vi "Configuration UI.vi"(0 "Engine":refnum<k7>, 5 "Data In":T1, 7 "Sequence Context In":refnum<k7>, 11 "error in (no error)":errorcluster) -> (4 "Engine out":refnum<k7>, 6 "Data Out":T1, 8 "Changed":bool, 15 "error out":errorcluster)   [LabVIEW 2019, in "STS_LTRV.lvlib"]
uses:
  STS_LTRV.lvlib
  TypeDefs/Config UI Data Type.ctl
  SimpleTextPlugin.llb/SimpleTextRpt - TestStand - End Modal Dialog (Engine).vi
  SimpleTextPlugin.llb/SimpleTextRpt - TestStand - Start Modal Dialog (Engine).vi
panel:
  in  "Max UUT Records to Store":u32=4 min=4
  in  "TS_HELP":bool
  in  "TS_CANCEL":bool
  in  "TS_OK":bool
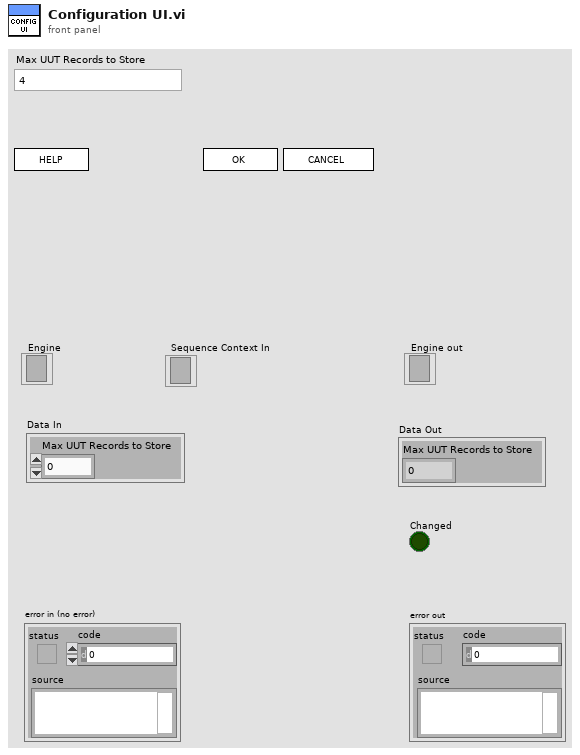
[diagram p1: front panel]
types:
  T1 = typedef "STS_LTRV.lvlib/Config UI Data Type.ctl" = cluster{"Max UUT Records to Store":u32}
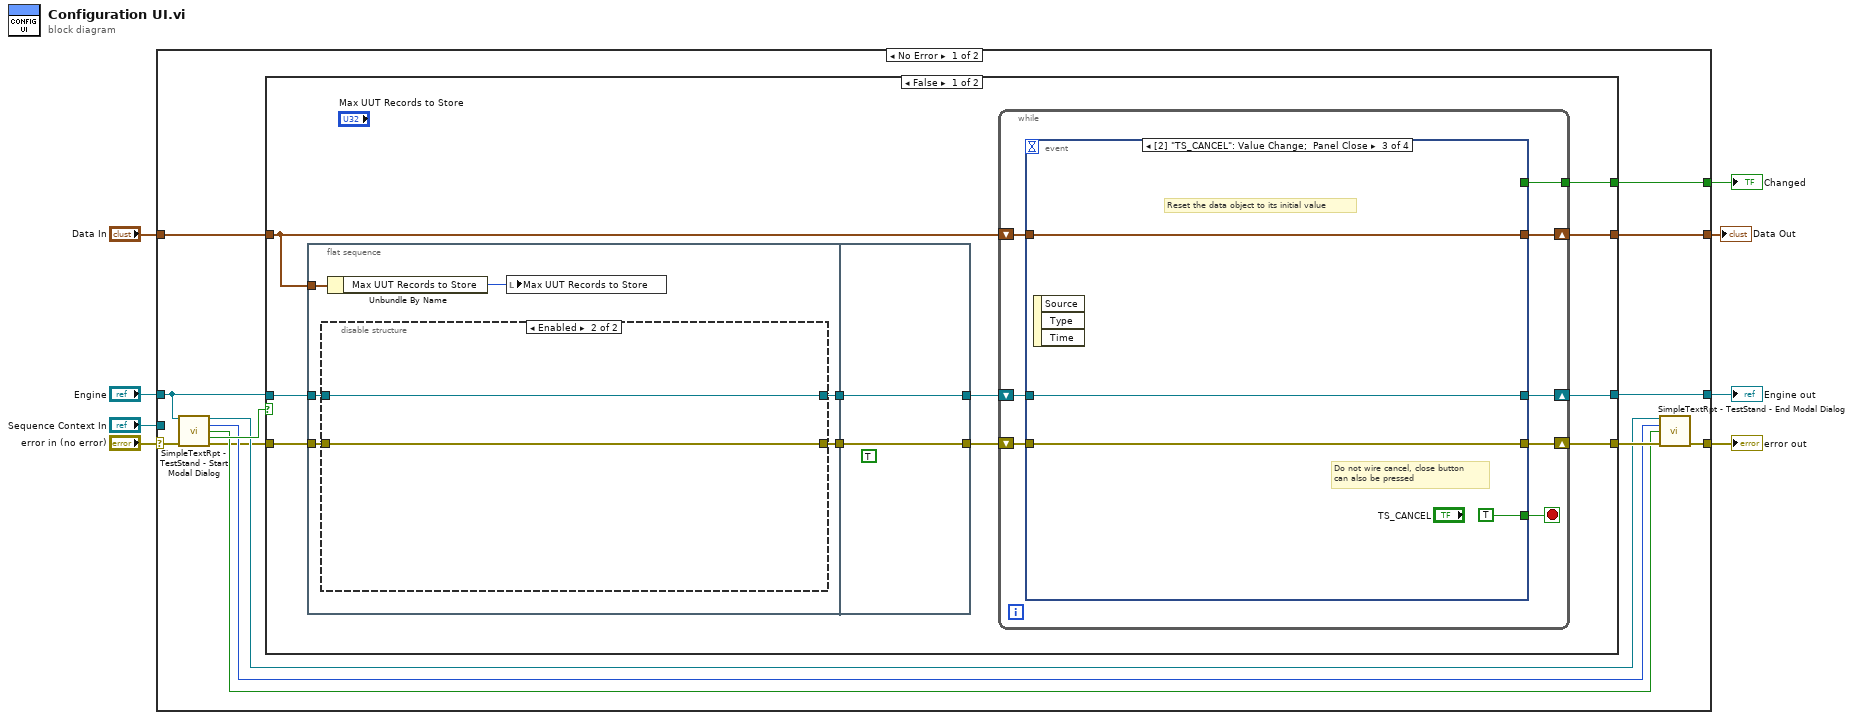
[diagram p0: block diagram]
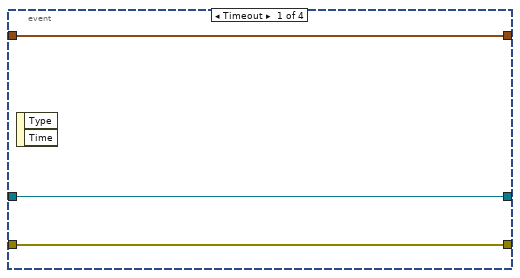
[diagram p2: hidden frame]
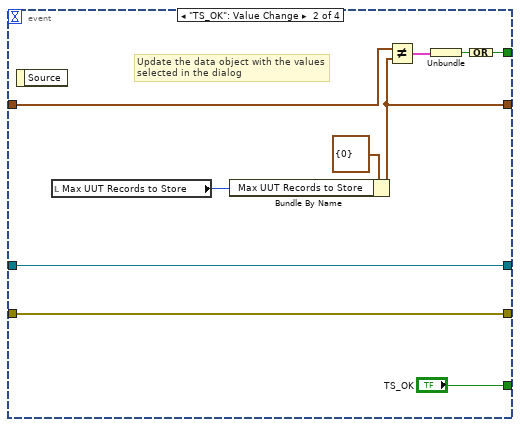
[diagram p3: hidden frame]
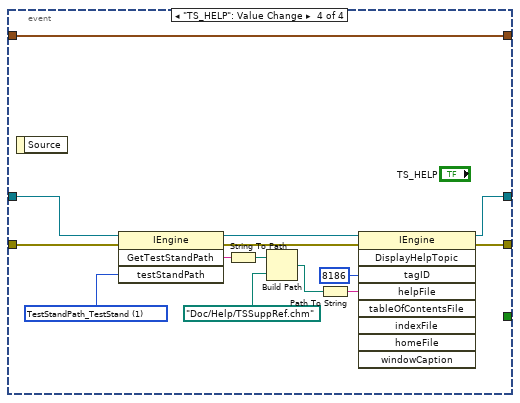
[diagram p4: hidden frame]
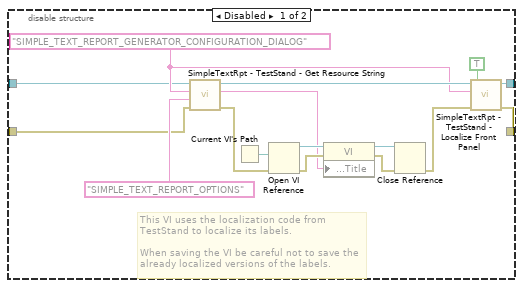
[diagram p5: hidden frame]
diagram:
  n1 = case shown="No Error" "error in (no error)" {
    selector: "error in (no error)" -> [w13 w103]
    tunnel: "Data In" -> [w21 w101]
    tunnel: [w18 w103] -> w7
    tunnel: [w14 w102] -> w3
    tunnel: [w15 _] -> w5
    tunnel: "Engine" -> [w11 w102]
    tunnel: "Sequence Context In" -> [_ _]
    tunnel: [w9 w101] -> w1
    frame No Error {
      n2 = call-poly "SimpleTextRpt - TestStand - Start Modal Dialog.vi"("Engine in"=w11, "error in (no error)"=w13) -> ("Engine out"=w12:refnum<k7>, "Modal ID"=w17:i32, "VI Originally Open"=w16:bool, "Should Abort"=w20:bool, "error out"=w10:errorcluster)  [unwired: 2 in, 7 out]
      n3 = case shown="False" w20 {
        tunnel: [w32 w100] -> w19
        tunnel: w21 -> [w30 w98]
        tunnel: w11 -> [w26 w99]
        tunnel: w10 -> [w24 w100]
        tunnel: [w29 _] -> w15
        tunnel: [w25 w99] -> w14
        tunnel: [w22 w98] -> w9
        frame False {
          n4 = flat-sequence {
            tunnel: w30 -> [w76]
            tunnel: w26 -> [w74]
            tunnel: [w77] -> w28
            tunnel: [w75] -> w27
            tunnel: w24 -> [w73]
            tunnel: [w97] -> w31
            tunnel: w28 -> [w97]
            tunnel: w27 -> [w96]
            tunnel: [w96] -> w23
            frame #0 {
              n5 = disable-structure shown="Enabled" {
                disable-tunnel: [w92 w94] -> w77
                disable-tunnel: [w91 w95] -> w75
                disable-tunnel: w74 -> [w79 w94]
                disable-tunnel: w73 -> [w78 w95]
                frame Disabled {
                  w85 = "SIMPLE_TEXT_REPORT_GENERATOR_CONFIGURATION_DIALOG" ("Category")
                  # "This VI uses the localization code from \nTestStand to localize its labels.\n\nWhen saving the VI be careful not to save the \nalready localized versions of the labels."
                  n6 = call "SimpleTextRpt - TestStand - Get Resource String.vi"("error in (no error)"=w78, "Symbol"="SIMPLE_TEXT_REPORT_OPTIONS", "Category"=w85, "Engine Reference In"=w79) -> ("error out"=w83:errorcluster, "Resource String"=w84:string, "Engine Reference Out"=w86:refnum<k7>)  [unwired: 4 in, 1 out]
                  n7 = Current VI's Path() -> (path=w90:path)
                  n8 = Open VI Reference(vi path=w90, error in (no error)=w83) -> (vi reference=w88:refnum<vi>, error out=w89:errorcluster)  [unwired: 4 in]
                  n9 = property class="VI"(reference=w88, error in=w89, "Front Panel.Title"=w84) -> (reference out=w80:refnum<vi>, error out=w87:errorcluster)
                  n10 = Close Reference(reference=w80, error in (no error)=w87) -> (error out=w81:errorcluster)
                  n11 = call "SimpleTextRpt - TestStand - Localize Front Panel.vi"("Engine Reference In"=w86, "Category"=w85, "error in (no error)"=w81, "Localize Free Labels (False)"=TRUE) -> ("Engine Reference Out"=w92:refnum<k7>, "error out"=w91:errorcluster)  [unwired: 1 in, 4 out]
                }
                frame Enabled {
                }
              }
              n12 = Unbundle By Name(w76) -> ("Max UUT Records to Store"=w72:u32)
              n13 = local write "Max UUT Records to Store"(w72) -> ()
            }
            frame #1 {
              (unwired) TRUE ("Selected")
            }
          }
          n14 = while {
            shift-right: [w39] -> w32
            shift-left: w23 -> [w38]
            shift-right: [w35] -> w25
            shift-left: w31 -> [w36]
            tunnel: [w34] -> w29
            shift-right: [w33] -> w22
            shift-left: w30 -> [w37]
            stop <- w40 stop-if-true
            n15 = event shown="[2] \"TS_CANCEL\": Value Change;  Panel Close" {
              selector: _ -> [_ _ _ _]
              dyn-events: _ -> [_ _ _ _]
              timeout: _ -> [_ _ _ _]
              tunnel: [_ "TS_OK" TRUE ("TS_OK") _] -> w40
              tunnel: [w43 w52 w57 w70] -> w39
              tunnel: w38 -> [w43 w52 w57 w66]
              tunnel: w37 -> [w41 w50 w54 w58]
              tunnel: w36 -> [w42 w51 w56 w68]
              tunnel: [w42 w51 w56 w69] -> w35
              tunnel: [_ w47 _ _] -> w34
              tunnel: [w41 w44 w54 w58] -> w33
              event Timeout {
                n16 = event-data() -> ()  [unwired: 3 out]
              }
              event "TS_OK": Value Change {
                # "Update the data object with the values \nselected in the dialog"
                n17 = event-data() -> ()  [unwired: 2 out]
                n18 = local read "Max UUT Records to Store"() -> (w45:u32)
                n19 = Bundle By Name(cluster=T1 {"Max UUT Records to Store"=0} ("Data In"), "Max UUT Records to Store"=w45) -> (w44:T1)
                n20 = Not Equal?(x=w50, y=w44) -> (x != y?=w49:cluster{"Max UUT Records to Store":bool})
                n21 = Unbundle(w49) -> ("Max UUT Records to Store"=w48:bool)
                n22 = Compound Arithmetic op=OR(w48) -> (w47:bool)
              }
              event "TS_CANCEL": Value Change; Panel Close {
                # "Do not wire cancel, close button\ncan also be pressed"
                # "Reset the data object to its initial value"
                n23 = event-data() -> ()  [unwired: 4 out]
              }
              event "TS_HELP": Value Change {
                w64 = 1 items=["TestStandPath_TestStand"=1, "TestStandPath_Bin"=2, "TestStandPath_Config"=3, "TestStandPath_Public"=4, "TestStandPath_CommonAppData"=5, "TestStandPath_LocalAppData"=6, "TestStandPath_PublicComponents"=7, "TestStandPath_NIComponents"=8, "TestStandPath_Temp"=9] ("testStandPath")
                n24 = event-data() -> ()  [unwired: 2 out]
                n25 = invoke class="IEngine" method="GetTestStandPath"(reference=w68, error in=w66, "testStandPath"=w64) -> (reference out=w67:refnum<k7>, error out=w65:errorcluster, "GetTestStandPath"=w62:string)  [unwired: 1 in, 1 out]
                n26 = String To Path(string=w62) -> (path=w63:path)
                n27 = Build Path(base path=w63, name or relative path=path "Doc/Help/TSSuppRef.chm") -> (appended path=w61:path)
                n28 = Path To String(path=w61) -> (string=w59:string)
                n29 = invoke class="IEngine" method="DisplayHelpTopic"(reference=w67, error in=w65, "tagID"=8186, "helpFile"=w59) -> (reference out=w69:refnum<k7>, error out=w70:errorcluster)  [unwired: 5 in, 7 out]
              }
            }
          }
        }
        frame True {
        }
      }
      n30 = call-poly "SimpleTextRpt - TestStand - End Modal Dialog.vi"("Engine"=w12, "Modal ID"=w17, "VI Originally Open"=w16, "error in (no error)"=w19) -> ("error out"=w18:errorcluster)  [unwired: 1 in, 10 out]
    }
    frame Error {
    }
  }
  "error out" <- w7
  "Changed" <- w5
  "Engine out" <- w3
  "Data Out" <- w1
